vi "RT Driver VI.vi"(7 "Operation":T1(ring), 11 "Device Reference in":u64 format="%.0x") -> (0 "Error Code":i32)   [LabVIEW 2026, in "Template Engine.lvlib"]
uses:
  Template Engine.lvlib
  <userlib>/Custom Device Interfaces_v1.lvlibp/Utility/Custom Device Utility.lvclass
  VS Custom Device API/NIVS Custom Device API.lvclass
  C:/Program Files/NI/LVAddons/nivscustomdeviceexpress/1/Targets/win64/user.lib/Custom Device Interfaces_v1.lvlibp/CustomDeviceAPI/Custom Device API.lvclass
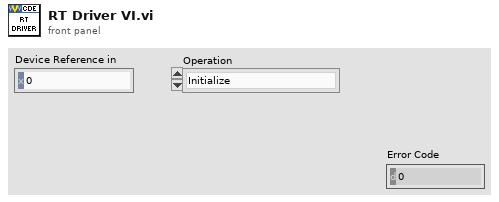
[diagram p1: front panel]
types:
  T1 = enum16{"Initialize", "Start", "Read Data from HW", "Write Data to HW", "Close"}
  T2 = cluster{"Custom Device Utility":refnum<class "Custom Device Utility.lvclass">, "NIVS Custom Device API":refnum<class "NIVS Custom Device API.lvclass">}
  T3 = cluster{"Name":string, "PPL Path":path, "Instance Name":string, "Compiled Settings":variant}
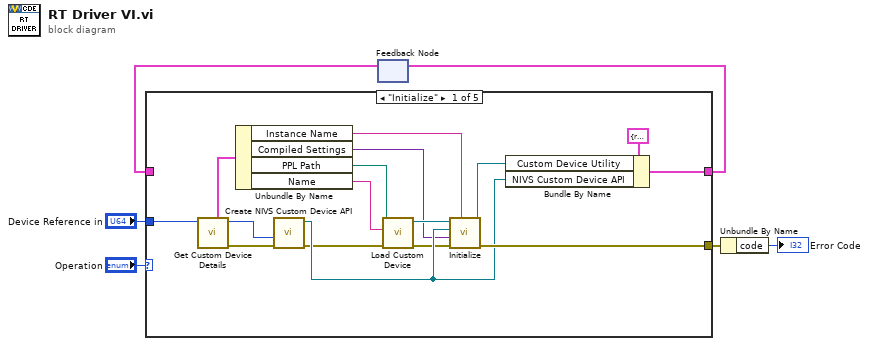
[diagram p0: block diagram]
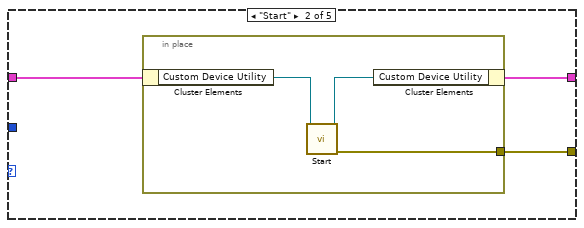
[diagram p2: hidden frame]
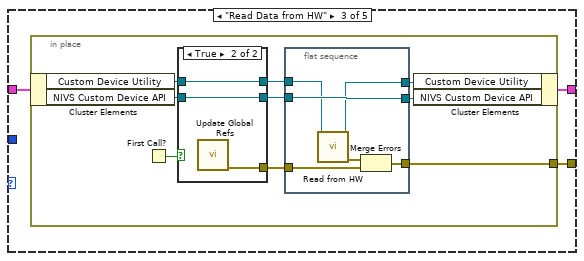
[diagram p3: hidden frame]
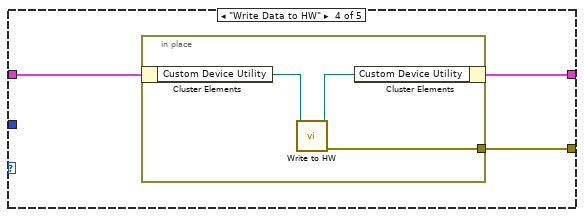
[diagram p5: hidden frame]
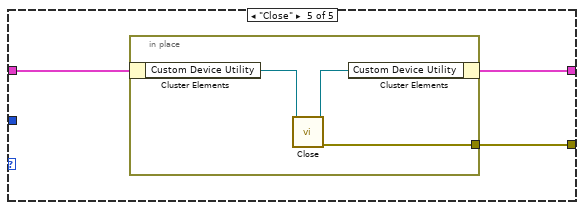
[diagram p6: hidden frame]
diagram:
  n1 = feedback #1() -> (w3:T2)  [unwired: 1 in]
  n2 = case shown="\"Initialize\"" "Operation" {
    tunnel: [w18 w24 w29 w52 w58] -> w4
    tunnel: w3 -> [_ w23 w30 w53 w59]
    tunnel: "Device Reference in" -> [w16 _ _ _ _]
    tunnel: [w22 w25 w31 w54 w60] -> w6
    frame "Initialize" {
      n3 = call "Get Custom Device Details.vi"("Device Reference in"=w16) -> ("error out"=w15:errorcluster, "Data Reference out"=w14:u64, "Custom Device Details"=w13:T3)  [unwired: 8 in]
      n4 = Unbundle By Name(w13) -> ("Instance Name"=w12:string, "Compiled Settings"=w11:variant, "PPL Path"=w8:path, "Name"=w7:string)
      n5 = call "Create NIVS Custom Device API.vi"("error in"=w15, "Custom Device Item Ref"=w14) -> ("error out"=w10:errorcluster, "NIVS Custom Device API out"=w17:refnum<class "NIVS Custom Device API.lvclass">)  [unwired: 8 in]
      n6 = call <userlib>:"Load Custom Device.vi"("error in"=w10, "Custom Device Name"=w7, "Path"=w8) -> ("error out"=w9:errorcluster, "Custom Device out"=w21:refnum<class "Custom Device.lvclass">)  [unwired: 7 in]
      n7 = call <userlib>:"Initialize.vi"("Custom Device in"=w21, "Custom Device Name"=w12, "error in"=w9, "Compiled Settings"=w11, "Custom Device API in"=w17) -> ("error out"=w22:errorcluster, "Custom Device Utility out"=w19:refnum<class "Custom Device Utility.lvclass">)  [unwired: 5 in]
      n8 = Bundle By Name(cluster=T2 {"Custom Device Utility"=refnum, "NIVS Custom Device API"=refnum}, "Custom Device Utility"=w19, "NIVS Custom Device API"=w17) -> (w18:T2)
    }
    frame "Start" {
      n9 = in-place {
        in-place-border: [w28] -> w25
        n10 = in-place-cluster #2(w23) -> ("Custom Device Utility"=w27:refnum<class "Custom Device Utility.lvclass">)
        n11 = call <userlib>:"Start.vi"("Custom Device Utility in"=w27) -> ("error out"=w28:errorcluster, "Custom Device Utility out"=w26:refnum<class "Custom Device Utility.lvclass">)  [unwired: 9 in]
        n12 = in-place-cluster #2("Custom Device Utility"=w26) -> (w24:T2)
      }
    }
    frame "Read Data from HW" {
      n13 = in-place {
        in-place-border: [w40] -> w31
        n14 = in-place-cluster #3(w30) -> ("Custom Device Utility"=w36:refnum<class "Custom Device Utility.lvclass">, "NIVS Custom Device API"=w37:refnum<class "NIVS Custom Device API.lvclass">)
        n15 = First Call?() -> (First Call?: T/F=w38:bool)
        n16 = case shown="True" w38 {
          tunnel: [_ w51] -> w39
          tunnel: w37 -> [w48 w50]
          tunnel: [w48 w50] -> w33
          tunnel: w36 -> [w47 w49]
          tunnel: [w47 w49] -> w35
          frame False {
          }
          frame True {
            n17 = call "Update Global Refs.vi"() -> ("error out"=w51:errorcluster)  [unwired: 11 in]
          }
        }
        n18 = flat-sequence {
          tunnel: [w45] -> w40
          tunnel: w39 -> [w44]
          tunnel: w35 -> [w41]
          tunnel: [w42] -> w34
          tunnel: w33 -> [w43]
          tunnel: [w43] -> w32
          frame #0 {
            n19 = call <userlib>:"Read from HW.vi"("Custom Device Utility in"=w41) -> ("error out"=w46:errorcluster, "Custom Device Utility out"=w42:refnum<class "Custom Device Utility.lvclass">)  [unwired: 9 in]
            n20 = Merge Errors(w46, w44) -> (w45:errorcluster)
          }
        }
        n21 = in-place-cluster #3("Custom Device Utility"=w34, "NIVS Custom Device API"=w32) -> (w29:T2)
      }
    }
    frame "Write Data to HW" {
      n22 = in-place {
        in-place-border: [w57] -> w54
        n23 = in-place-cluster #4(w53) -> ("Custom Device Utility"=w56:refnum<class "Custom Device Utility.lvclass">)
        n24 = call <userlib>:"Write to HW.vi"("Custom Device Utility in"=w56) -> ("error out"=w57:errorcluster, "Custom Device Utility out"=w55:refnum<class "Custom Device Utility.lvclass">)  [unwired: 9 in]
        n25 = in-place-cluster #4("Custom Device Utility"=w55) -> (w52:T2)
      }
    }
    frame "Close" {
      n26 = in-place {
        in-place-border: [w63] -> w60
        n27 = in-place-cluster #5(w59) -> ("Custom Device Utility"=w62:refnum<class "Custom Device Utility.lvclass">)
        n28 = call <userlib>:"Close.vi"("Custom Device Utility in"=w62) -> ("error out"=w63:errorcluster, "Custom Device Utility out"=w61:refnum<class "Custom Device Utility.lvclass">)  [unwired: 9 in]
        n29 = in-place-cluster #5("Custom Device Utility"=w61) -> (w58:T2)
      }
    }
  }
  n30 = feedback-in #1(w4) -> ()
  n31 = Unbundle By Name(w6) -> ("code"=→"Error Code":i32)
